vi "Projection-Frustum.vi"(4 "Far Clipping Plane":sgl, 5 "Near Clipping Plane":sgl, 6 "Top":sgl, 7 "Bottom":sgl, 8 "error in (no error)":errorcluster, 9 "Right":sgl, 10 "Left":sgl, 11 "SceneGraphDisplay in":refnum<class "SceneGraphDisplay.lvclass">) -> (0 "error out":errorcluster, 3 "SceneGraphDisplay out":refnum<class "SceneGraphDisplay.lvclass">)   [LabVIEW 2015, in "SceneGraphDisplay.lvclass"]
doc: "Sets coordinates to render the scene in a frustum-shaped view. This projection causes objects farther from the camera to appear smaller.\n\nQControl Class wrapper around the <b>SceneGraphDisplay : Projection:Frustum Method</b>.\n<b> </b> <b> </b>\n©2016 Q Software Innovations, LLC (QSI)\nwritten by Quentin Alldredge\nproduced in LabVIEW 2015\n\nsupport@qsoftwareinnovations.com\nwww.qsoftwareinnovations.com\n\nAll rights reserved.\n\nRedistribution and use in source and binary forms, with or without modification, are permitted provided that the following conditions are met:\n\n * Redistributions of source code must retain the above copyright notice, this list of conditions and the following disclaimer.\n * Redistributions in binary form must reproduce the above copyright notice, this list of conditions and the following disclaimer in the documentation and/or other materials provided with the distribution.\n * Neither the name of Q Software Innovations, LLC. nor the names of its contributors may be used to endorse or promote products derived from this software without specific prior written permission.\n\nTHIS SOFTWARE IS PROVIDED BY THE COPYRIGHT HOLDERS AND CONTRIBUTORS \"AS IS\" AND ANY EXPRESS OR IMPLIED WARRANTIES, INCLUDING, BUT NOT LIMITED TO, THE IMPLIED WARRANTIES OF MERCHANTABILITY AND FITNESS FOR A PARTICULAR PURPOSE ARE DISCLAIMED. IN NO EVENT SHALL THE COPYRIGHT OWNER OR CONTRIBUTORS BE LIABLE FOR ANY DIRECT, INDIRECT, INCIDENTAL, SPECIAL, EXEMPLARY, OR CONSEQUENTIAL DAMAGES (INCLUDING, BUT NOT LIMITED TO, PROCUREMENT OF SUBSTITUTE GOODS OR SERVICES; LOSS OF USE, DATA, OR PROFITS; OR BUSINESS INTERRUPTION) HOWEVER CAUSED AND ON ANY THEORY OF LIABILITY, WHETHER IN CONTRACT, STRICT LIABILITY, OR TORT (INCLUDING NEGLIGENCE OR OTHERWISE) ARISING IN ANY WAY OUT OF THE USE OF THIS SOFTWARE, EVEN IF ADVISED OF THE POSSIBILITY OF SUCH DAMAGE."
uses:
  SceneGraphDisplay.lvclass
  SceneGraphDisplay.lvclass/SceneGraphDisplay.ctl
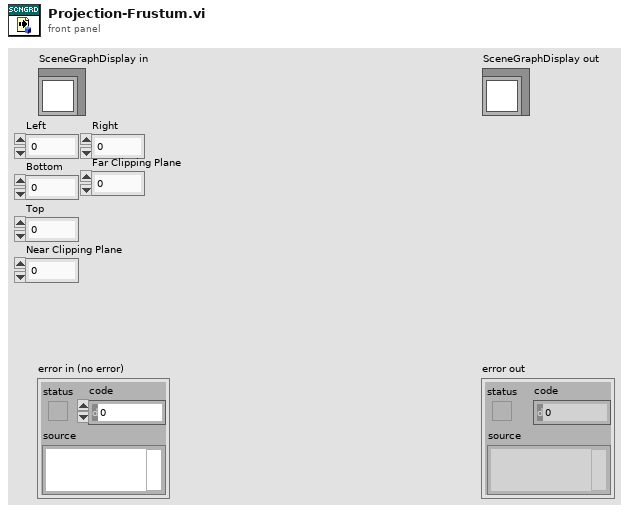
[diagram p1: front panel]
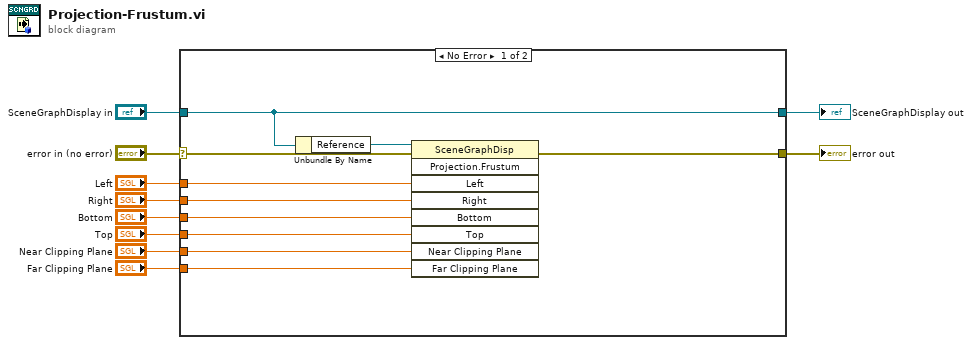
[diagram p0: block diagram]
diagram:
  n1 = case shown="No Error" "error in (no error)" {
    selector: "error in (no error)" -> [w20 w22]
    tunnel: [w19 w22] -> w9
    tunnel: [w18 w21] -> w7
    tunnel: "SceneGraphDisplay in" -> [w18 w21]
    tunnel: "Left" -> [w16 _]
    tunnel: "Right" -> [w15 _]
    tunnel: "Bottom" -> [w14 _]
    tunnel: "Top" -> [w13 _]
    tunnel: "Near Clipping Plane" -> [w12 _]
    tunnel: "Far Clipping Plane" -> [w11 _]
    frame No Error {
      n2 = Unbundle By Name(w18) -> ("Reference"=w17:refnum<vi>)
      n3 = invoke class="SceneGraphDisp" method="Projection.Frustum"(reference=w17, error in=w20, "Left"=w16, "Right"=w15, "Bottom"=w14, "Top"=w13, "Near Clipping Plane"=w12, "Far Clipping Plane"=w11) -> (error out=w19:errorcluster)  [unwired: 1 in, 8 out]
    }
    frame Error {
    }
  }
  "error out" <- w9
  "SceneGraphDisplay out" <- w7
